vi "Actor Core.vi"(8 "error in":errorcluster, 11 "Nested in":refnum<class "Nested Actor.lvclass">) -> (0 "error out":errorcluster, 3 "Actor out":refnum<class "Actor.lvclass">)   [LabVIEW 2020, in "Nested Actor.lvlib" / "Nested Actor.lvclass"]
doc: "(<B>Filename</B>: Actor Framework.lvlib:Actor.lvclass:Actor Core.vi)\n\nReceives messages to the actor, reacts to them, and initiates any error handling that may shut the actor down.\n\nDescendant classes may override this VI to append parallel tasks for the actor to complete while it handles messages. Overrides use the Call Parent Method node."
uses:
  Nested Actor.lvclass
  C:/Program Files (x86)/National Instruments/LabVIEW 2020/vi.lib/ActorFramework/Actor/Actor.lvclass
  <vilib>/ActorFramework/Actor/Actor.lvclass
  <vilib>/ActorFramework/Actor/Actor.lvclass/Actor.ctl
  <vilib>/ActorFramework/Message Enqueuer/Message Enqueuer.lvclass/Message Enqueuer.ctl
  Nested Actor.lvclass/Nested Actor.ctl
  Nested Actor Messages/Abstract Message Msg/Abstract Message Msg.lvclass/Abstract Message Msg.ctl
  <vilib>/ActorFramework/Message Enqueuer/Init from Existing Queue.vi
  <vilib>/ActorFramework/Message Enqueuer/Enqueue.vi
  <vilib>/ActorFramework/Stop Msg/Stop Msg.lvclass
  C:/Program Files (x86)/National Instruments/LabVIEW 2020/vi.lib/ActorFramework/Message/Message.lvclass
  Nested Actor Messages/Abstract Message Msg/Abstract Message Msg.lvclass
  Interface Message Specifier Messages/Save Buffered Data Msg/Save Buffered Data Msg.lvclass
  <vilib>/ActorFramework/Message Priority Queue/Priority Enqueue.vi
  <vilib>/ActorFramework/Message Enqueuer/Message Enqueuer.lvclass
panel:
  in  "Send Interface Message":bool
  in  "Send Abstract Message":bool
  out "Actor Type":string
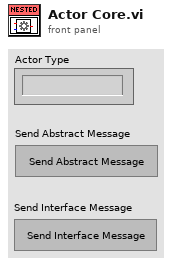
[diagram p1: front panel]
types:
  T1 = typedef "Nested Actor.lvlib/Nested Actor.lvclass/Actor Type.ctl" = enum16{"Slow Buffer", "Fast Buffer"}
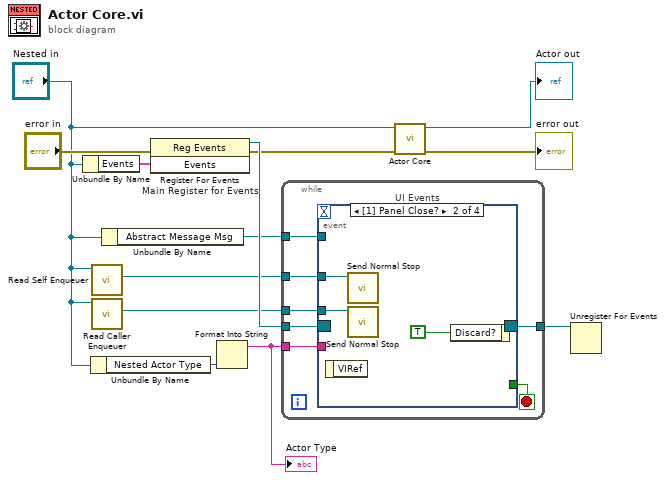
[diagram p0: block diagram]
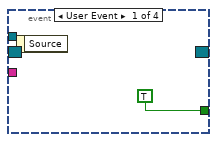
[diagram p2: hidden frame]
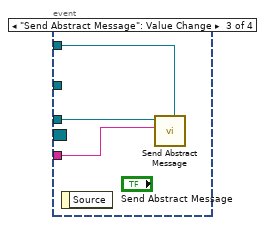
[diagram p3: hidden frame]
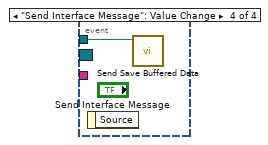
[diagram p4: hidden frame]
diagram:
  n1 = Unbundle By Name("Nested in") -> ("Events"=w10:cluster{"Stop":refnum<user-event>})
  n2 = Unbundle By Name("Nested in") -> ("Nested Actor Type"=w5:T1)
  n3 = call <vilib>:"Read Self Enqueuer.vi"("Actor"="Nested in") -> ("Self Enqueuer"=w8:refnum<class "Message Enqueuer.lvclass">)  [unwired: 10 in]
  n4 = call <vilib>:"Read Caller Enqueuer.vi"("Actor"="Nested in") -> ("Caller Enqueuer"=w2:refnum<class "Message Enqueuer.lvclass">)  [unwired: 10 in]
  n5 = Unbundle By Name("Nested in") -> ("Abstract Message Msg"=w4:refnum<class "Abstract Message Msg.lvclass">)
  n6 = register-events "Main Register for Events"(error in="error in", w10) -> (reference out=w11:refnum<event-registration>, error out=w6:errorcluster)  [unwired: 1 in]
  n7 = Format Into String(w5) -> (resulting string=w1:string)  [unwired: 3 in, 1 out]
  "Actor Type" <- w1
  n8 = while {
    tunnel: w11 -> [w20]
    tunnel: [w18] -> w9
    tunnel: w8 -> [w17]
    tunnel: w4 -> [w16]
    tunnel: w2 -> [w15]
    tunnel: w1 -> [w14]
    stop <- w19 stop-if-true
    n9 = event "UI Events" shown="[1] Panel Close?" {
      selector: w20 -> [_ _ _ _]
      dyn-events: [_ _ _ _] -> w18
      timeout: _ -> [_ _ _ _]
      tunnel: [TRUE _ _ _] -> w19
      tunnel: w17 -> [_ w23 _ _]
      tunnel: w16 -> [_ _ w27 _]
      tunnel: w15 -> [_ w22 w26 w28]
      tunnel: w14 -> [_ _ w25 _]
      event User Event {
        n10 = event-data() -> ()  [unwired: 1 in, 1 out]
      }
      event Panel Close? {
        n11 = event-data() -> ()  [unwired: 1 in, 1 out]
        n12 = call <vilib>:"Send Normal Stop.vi"("Message Enqueuer"=w23) -> ()  [unwired: 10 in, 1 out]
        n13 = call <vilib>:"Send Normal Stop.vi"("Message Enqueuer"=w22) -> ()  [unwired: 10 in, 1 out]
        n14 = event-data("Discard?"=TRUE) -> ()  [unwired: 1 in, 1 out]
      }
      event "Send Abstract Message": Value Change {
        n15 = event-data() -> ()  [unwired: 1 in, 1 out]
        n16 = call "Send Abstract Message.vi"("Message Type"=w27, "Msg Data String"=w25, "Message Enqueuer"=w26) -> ()  [unwired: 7 in, 2 out]
      }
      event "Send Interface Message": Value Change {
        n17 = event-data() -> ()  [unwired: 1 in, 1 out]
        n18 = call "Send Save Buffered Data.vi"("Message Enqueuer"=w28) -> ()  [unwired: 9 in, 2 out]
      }
    }
  }
  n19 = call-parent "Actor Core.vi"("error in"=w6, "Actor in"="Nested in") -> ("error out"=→"error out":errorcluster, "Actor out"=→"Actor out":refnum<class "Actor.lvclass">)  [unwired: 8 in]
  n20 = Unregister For Events(event registration refnum=w9) -> ()  [unwired: 1 in, 1 out]
